vi "grSim Command.vi"(8 "FIRASim?":bool=TRUE, 9 "Robots":T1[](array[typedef]), 10 "isteamyellow":bool=TRUE, 11 "timestamp":dbl format="%#_13g") -> (1 "Command":u8[](array[numeric]))   [LabVIEW 2023]
uses:
  Convert AI Robot to Robot Command Folder/grSim/grSim Robot Command.ctl
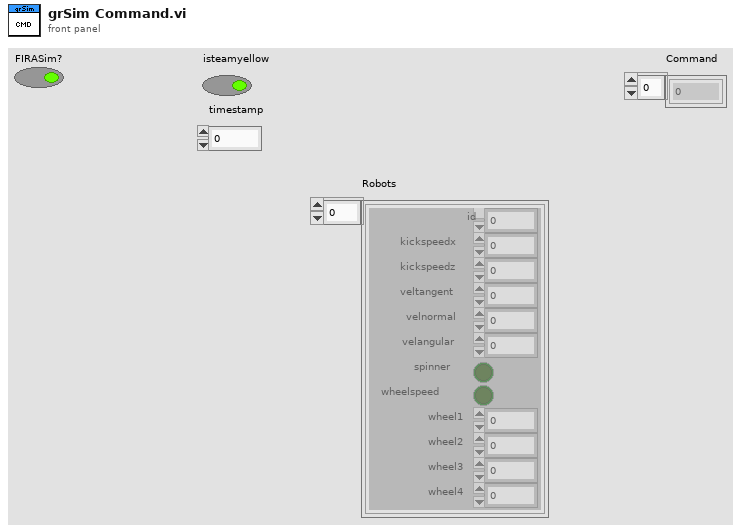
[diagram p1: front panel]
types:
  T1 = typedef "grSim Robot Command.ctl" = cluster{"id":u32, "kickspeedx":sgl, "kickspeedz":sgl, "veltangent":sgl, "velnormal":sgl, "velangular":sgl, "spinner":bool, "wheelspeed":bool, "wheel1":sgl, "wheel2":sgl, "wheel3":sgl, "wheel4":sgl}
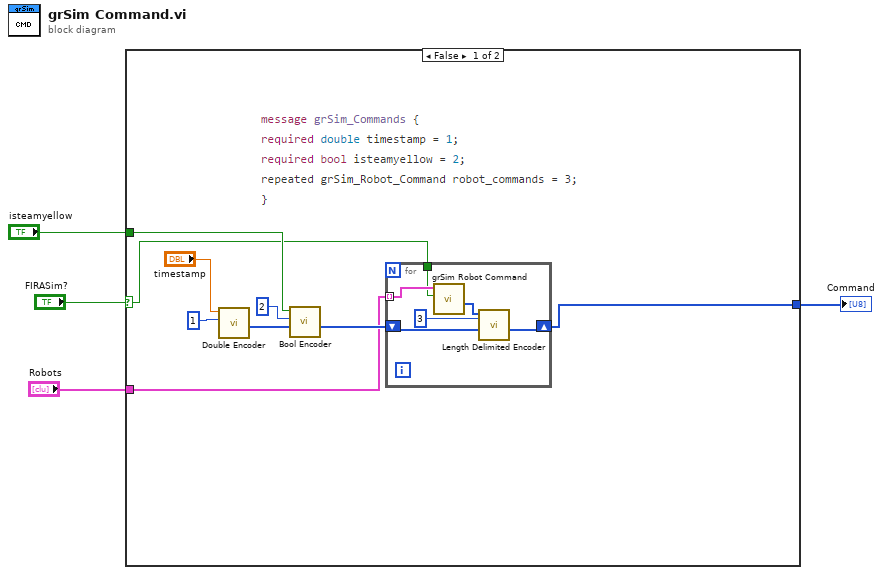
[diagram p0: block diagram]
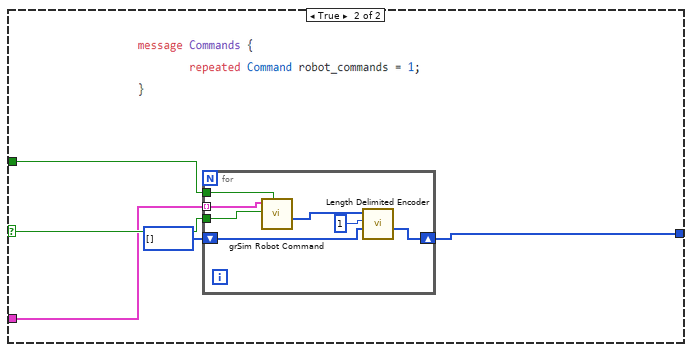
[diagram p2: hidden frame]
diagram:
  n1 = case shown="False" "FIRASim?" {
    selector: "FIRASim?" -> [w5 w23]
    tunnel: "isteamyellow" -> [w8 w22]
    tunnel: "Robots" -> [w7 w21]
    tunnel: [w6 w24] -> w1
    frame False {
      n2 = call "Double Encoder.vi"("Key"=u32 1, "Value"="timestamp") -> ("Array"=w12:u8[])  [unwired: 9 in]
      n3 = call "Bool Encoder.vi"("Array In"=w12, "Key"=u32 2, "Value"=w8) -> ("Array"=w9:u8[])  [unwired: 8 in]
      n4 = for {
        shift-right: [w16] -> w6
        shift-left: w9 -> [w17]
        tunnel: w7 -> [w19] mode=indexing
        tunnel: w5 -> [w14]
        n5 = call "grSim Robot Command.vi"("FIRASim?"=w14, "Robots"=w19) -> ("Array"=w18:u8[])  [unwired: 9 in]
        n6 = call "Length Delimited Encoder.vi"("Array In"=w17, "Key"=u32 3, "Array In 2"=w18) -> ("Array"=w16:u8[])  [unwired: 8 in]
      }
    }
    frame True {
      n7 = for {
        tunnel: w22 -> [w30]
        shift-right: [w31] -> w24
        shift-left: u8[] [] ("Array") -> [w26]
        tunnel: w21 -> [w27] mode=indexing
        tunnel: w23 -> [w25]
        n8 = call "grSim Robot Command.vi"("YellowTeam?"=w30, "FIRASim?"=w25, "Robots"=w27) -> ("Array"=w28:u8[])  [unwired: 8 in]
        n9 = call "Length Delimited Encoder.vi"("Array In"=w26, "Key"=u32 1, "Array In 2"=w28) -> ("Array"=w31:u8[])  [unwired: 8 in]
      }
    }
  }
  "Command" <- w1
